vi "Get TDMSState.vi"(8 "error in (no error)":errorcluster, 11 "Log_Engine in":refnum<class "Log_Engine.lvclass">) -> (0 "error out":errorcluster, 2 "TDMSState":T1, 3 "Log_Engine out":refnum<class "Log_Engine.lvclass">)   [LabVIEW 2019, in "Log_Engine.lvclass"]
doc: "Developed by Kevin Thompson\nkevin@thompsonengineering.net\n\nCopyright 2018\nThompson Engineering, LLC"
uses:
  Log_Engine.lvclass
  Common/DataTypes/TDMSState--enum.ctl
  Log_Engine.lvclass/Log_Engine.ctl
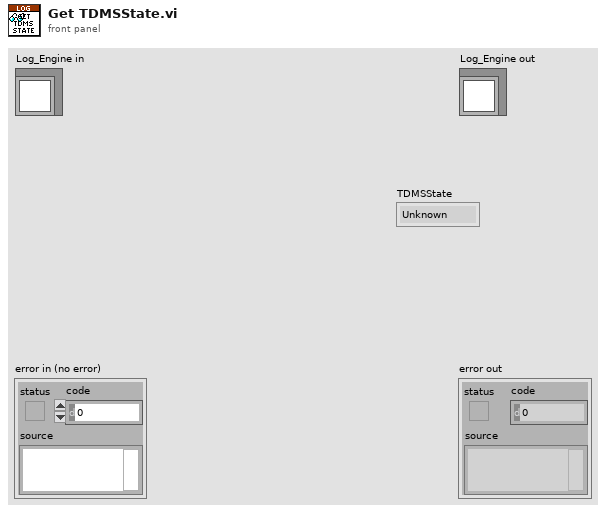
[diagram p1: front panel]
types:
  T1 = typedef "TDMSState--enum.ctl" = enum16{"Unknown", "Stopped", "Running", "Error"}
  T2 = typedef "Log_Engine.lvclass/ObjData--cluster.ctl" = cluster{"Settings":T3, "Public Events":T4, "Dependency":T5, "ReadData-placeholder":T6, "VISA-placeholder":refnum<visa-resource-name>, "InverterWaveformsQ":T7, "LogState":T8, "TDMSState":T1}
  T3 = typedef "Log_Engine.lvclass/Settings--cluster.ctl" = cluster{"Simulation":bool, "TDMS_FolderPath":string, "CSV_FolderPath":string, "TDMS_FileName_Prefix":string, "CSV_FileName_Prefix":string, "TDMS_LogDuration(s)":dbl, "CSV_LogDuration(s)":dbl}
  T4 = typedef "Log_Engine.lvclass/Public Events--cluster.ctl" = cluster{"Log_Engine.AsyncCmd Event":refnum<user-event>, "Log_Engine.AsyncMsg Event":refnum<user-event>, "stop process":refnum<user-event>, "Log_Engine.LogStateChg Ev":refnum<user-event>, "Log_Engine.TDMSStateChg Ev":refnum<user-event>}
  T5 = typedef "Log_Engine.lvclass/Dependency--cluster.ctl" = cluster{"Config":refnum<class "Config.lvclass">, "DAQ_Engine":refnum<class "DAQ_Engine.lvclass">}
  T6 = typedef "Log_Engine.lvclass/Read Data--cluster.ctl" = cluster{"Data":dbl}
  T7 = typedef "InverterWaveforms--QRef.ctl" = refnum<queue>
  T8 = typedef "LogState--enum.ctl" = enum16{"Unknown", "Stopped", "Running", "Error"}
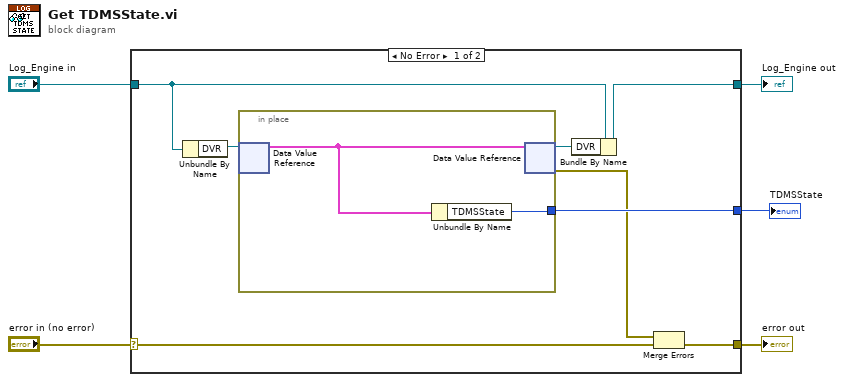
[diagram p0: block diagram]
diagram:
  n1 = case shown="No Error" "error in (no error)" {
    selector: "error in (no error)" -> [w13 w16]
    tunnel: [w7 w16] -> w4
    tunnel: [w9 w17] -> w2
    tunnel: "Log_Engine in" -> [w10 w17]
    tunnel: [w8 _] -> w1
    frame No Error {
      n2 = Unbundle By Name(w10) -> ("DVR"=w11:refnum<data-value>)
      n3 = in-place {
        in-place-border: [w14] -> w8
        n4 = in-place-dvr #1(w11) -> (w15:T2)  [unwired: 1 out]
        n5 = Unbundle By Name(w15) -> ("TDMSState"=w14:T1)
        n6 = in-place-dvr #1(w15) -> (w12:refnum<data-value>, w6:errorcluster)
      }
      n7 = Bundle By Name(cluster=w10, "DVR"=w12) -> (w9:refnum<class "Log_Engine.lvclass">)
      n8 = Merge Errors(w6, w13) -> (w7:errorcluster)
    }
    frame Error {
    }
  }
  "error out" <- w4
  "Log_Engine out" <- w2
  "TDMSState" <- w1
